vi "Initialize (Reference).vi"(8 "error in (no error)":errorcluster, 11 "FPGA Refnum":refnum<k20>) -> (0 "error out":errorcluster, 3 "FPGA Interface out":refnum<class "FPGA Interface.lvclass">)   [LabVIEW 2016, in "BCI-1553 API.lvlib" / "FPGA Interface.lvlib" / "FPGA Interface.lvclass"]
doc: "Initializes the resources for a bitfile that has already been setup for use with the BCI-1553 modules."
uses:
  FPGA Interface.lvclass
  <vilib>/rvi/interface/nirviMethod/nirviMethod.xnode
  <vilib>/FPGAPlugInAG/Dynamic/niLvFpga_ConfigureFifo_Dynamic.vi
  <vilib>/rvi/errors/niLvFpgaMergeErrorWithErrorCode.vi
  <vilib>/FPGAPlugInAG/Dynamic/niLvFpga_ReadFifo_Dynamic.vi
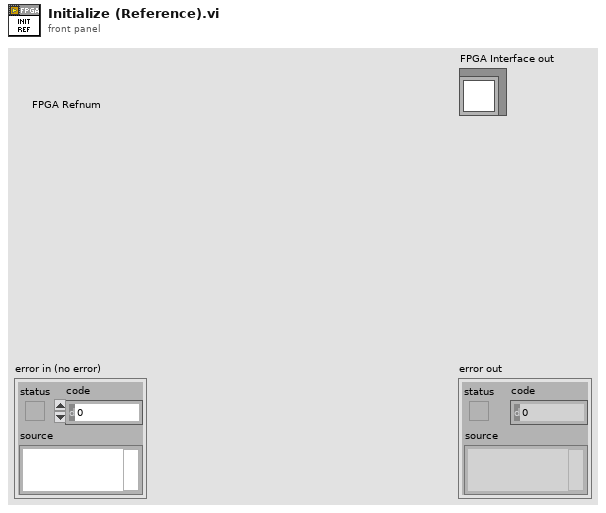
[diagram p1: front panel]
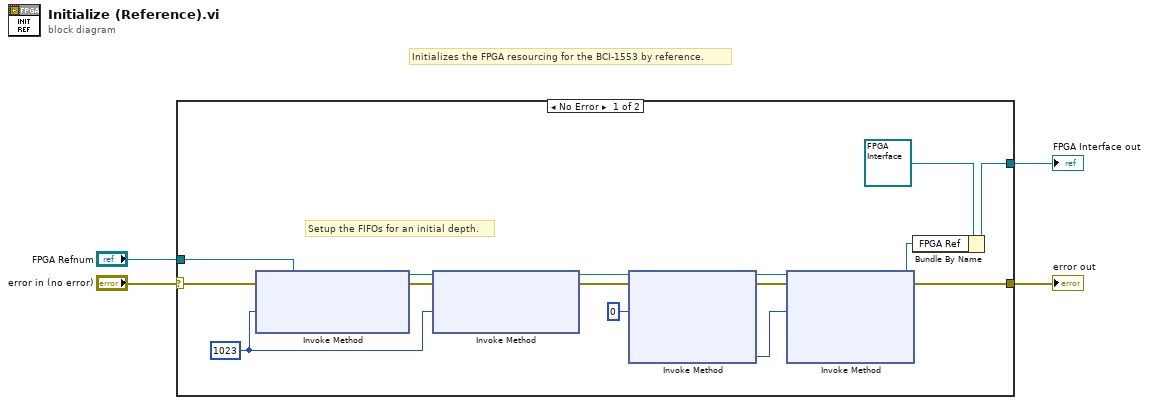
[diagram p0: block diagram]
diagram:
  # "Initializes the FPGA resourcing for the BCI-1553 by reference."
  n1 = case shown="No Error" "error in (no error)" {
    selector: "error in (no error)" -> [w5 w20]
    tunnel: [w9 w20] -> w1
    tunnel: [w18 _] -> w2
    tunnel: "FPGA Refnum" -> [w6 _]
    frame No Error {
      w15 = u32 1023 ("Requested Depth")
      # "Setup the FIFOs for an initial depth."
      n2 = xnode "Invoke Method"("FPGA VI Reference In"=w6, "error in"=w5, "Requested Depth"=w15) -> ("FPGA VI Reference Out"=w17:refnum<k20>, "error out"=w16:errorcluster)  [unwired: 1 out]
      n3 = xnode "Invoke Method"("FPGA VI Reference In"=w17, "error in"=w16, "Requested Depth"=w15) -> ("FPGA VI Reference Out"=w11:refnum<k20>, "error out"=w8:errorcluster)  [unwired: 1 out]
      n4 = xnode "Invoke Method"("FPGA VI Reference In"=w11, "error in"=w8, "Number of Elements"=u32 0) -> ("FPGA VI Reference Out"=w12:refnum<k20>, "error out"=w7:errorcluster, "Elements Remaining"=w13:u32)  [unwired: 1 in, 1 out]
      n5 = xnode "Invoke Method"("FPGA VI Reference In"=w12, "error in"=w7, "Number of Elements"=w13) -> ("FPGA VI Reference Out"=w10:refnum<k20>, "error out"=w9:errorcluster)  [unwired: 1 in, 2 out]
      n6 = Bundle By Name(cluster=refnum<class "FPGA Interface.lvclass"> refnum ("FPGA Interface in"), "FPGA Ref"=w10) -> (w18:refnum<class "FPGA Interface.lvclass">)
    }
    frame Error {
    }
  }
  "error out" <- w1
  "FPGA Interface out" <- w2
